vi "read All reg.vi"() -> ()   [LabVIEW 2010]
panel:
  out "x-y":u32=20388
  out "Array 2":i16[](array[numeric])=[5270, 1, 6098, 0, 2200, 2310, 7, 8, 8, 3, 3, 3, 3, 0, 0, -32000, 14, 30, 0, 0, 0, 0, 0, 0, 0, 0, 0, 0, 0, 0, 1, 0, 0, 0, 0, 0, 1, -32000, 0, 0, 0, 0, 1, 0, 0, 0, 0, 1, 0, 0, 0, -1, -999, -999, -999, 999, 999, 999, 90, 0, 0, 24, 0, 0, 0, -1, -999, -999, -999, 999, 999, 999, 90, 0, 24, 0, 0, 0, 0, 0, 14, 0, 0, 0, 0, 0, 10, 2, 1, 14, 0, 0, 0, 0, 0, 2, 14, 0, 0, 0, 0, 0, 2, 1, 1, 1, 1, 1, 1, 2, 14, 0, 0, 0, 0, 0, 2, 14, 0, 0, 0, 0, 0, 10, 2, 1, 14, 0, 0, 0, 0, 0, 2, 14, 0, 0, 0, 0, 0, 2, 14, 0, 0, 0, 0, 0, 2, 14, 0, 0, 0, 0, 0, 2, 0, 0, 0, 815, 0, 0, 0, 0, 0, 4, 0, 0, 815, 0, 0, 0, 0, 0, 4, 0, 0, 815, 0, 0, 0, 0, 0, 32, 1500, 32, 1500, 32, 1500, 1, 0, 0, 2, 0, 0, 0, 0, 0, 0, 0, 816, 0, 100, 0, 0, 0, 0, 0, 2, 0, 0, 0, 0, 0, 0, 0, 816, 0, 100, 0, 0, 1, 0, 100, 0, 0, 0, 100, 0, 0, 0, 0, 1, 0, 0, 0, 0, 0, 0, 0, 0, 0, 0, 0, 0, -1, -1, -1, -1, -1, -1, -1, -1, 1, 0, 0, 0, 1, 10, 0, 39, 239, 0, 1, 0, 0, 0, 0, 0, 0, 0, 0, 70, 52, 70, 52, 15, 16, 2, 4, 5, 22, 23, 24, 21, 14, 12, 13, 6, 7, 11, 10, 954, 12816, 13472, 0, 0, -32000, -32000, -32000, 50, 0, 21, 8, 24, 6, 28, 2011, 0, 1, 0, -19999, -19999, 9999, 9999, 0, 0, 0, 0, 0, 0, 0, 0, 0, 0, 0, 0, 0, 100, 30, 0, 0, -100, 30, 0, 0, 0, 0, 30, 10, 14, 0, 0, 0, 0, 0, 10, 2, 1, 14, 0, 0, 0, 0, 0, 2, 14, 0, 0, 0, 0, 0, 2, 14, 0, 0, 0, 0, 0, 2, 14, 0, 0, 0, 0, 0, 2, 14, 0, 0, 0, 0, 0, 10, 2, 1, 14, 0, 0, 0, 0, 0, 2, 14, 0, 0, 0, 0, 0, 2, 14, 0, 0, 0, 0, 0, 2, 14, 0, 0, 0, 0, 0, 2, 25, 0, 0, 0, 0, 0, 3, 25, 0, 0, 0, 0, 0, 3, 25, 0, 0, 0, 0, 0, 3, 25, 0, 0, 0, 0, 0, 3, 25, 0, 0, 0, 0, 0, 3, 25, 0, 0, 0, 0, 0, 3, 25, 0, 0, 0, 0, 0, 3, 25, 0, 0, 0, 0, 0, 3, 25, 0, 0, 0, 0, 0, 3, 25, 0, 0, 0, 0, 0, 3, 56, 55, 56, 55, 56, 56, 56, 78, 49, 32, 68, 73, 71, 73, 84, 32, 73, 78, 50, 32, 68, 73, 71, 73, 84, 32, 73, 78, 51, 32, 68, 73, 71, 73, 84, 32, 73, 78, 52, 32, 68, 73, 71, 73, 84, 32, 79, 85, 84, 49, 68, 73, 71, 73, 84, 32, 79, 85, 84, 50, 68, 73, 71, 73, 84, 32, 79, 85, 84, 51, 68, 73, 71, 73, 84, 32, 79, 85, 84, 52, 68, 73, 71, 73, 84, 32, 79, 85, 84, 53, 68, 73, 71, 73, 84, 32, 79, 85, 84, 54, 68, 73, 71, 73, 84, 32, 79, 85, 84, 55, 68, 73, 71, 73, 84, 32, 79, 85, 84, 56, 65, 76, 65, 82, 77, 49, 32, 32, 32, 32, 65, 76, 65, 82, 77, 50, 32, 32, 32, 32, 80, 82, 79, 70, 73, 76, 69, 49, 32, 32, 80, 82, 79, 70, 73, 76, 69, 50, 32, 32, 80, 82, 79, 70, 73, 76, 69, 51, 32, 32, 80, 82, 79, 70, 73, 76, 69, 52, 32, 32, 80, 82, 79, 70, 73, 76, 69, 53, 32, 32, 80, 82, 79, 70, 73, 76, 69, 54, 32, 32, 80, 82, 79, 70, 73, 76, 69, 55, 32, 32, 80, 82, 79, 70, 73, 76, 69, 56, 32, 32, 80, 82, 79, 70, 73, 76, 69, 57, 32, 32, 80, 82, 79, 70, 73, 76, 69, 49, 48, 32, 80, 82, 79, 70, 73, 76, 69, 49, 49, 32, 80, 82, 79, 70, 73, 76, 69, 49, 50, 32, 80, 82, 79, 70, 73, 76, 69, 49, 51, 32, 80, 82, 79, 70, 73, 76, 69, 49, 52, 32, 80, 82, 79, 70, 73, 76, 69, 49, 53, 32, 80, 82, 79, 70, 73, 76, 69, 49, 54, 32, 80, 82, 79, 70, 73, 76, 69, 49, 55, 32, 80, 82, 79, 70, 73, 76, 69, 49, 56, 32, 80, 82, 79, 70, 73, 76, 69, 49, 57, 32, 80, 82, 79, 70, 73, 76, 69, 50, 48, 32, 80, 82, 79, 70, 73, 76, 69, 50, 49, 32, 80, 82, 79, 70, 73, 76, 69, 50, 50, 32, 80, 82, 79, 70, 73, 76, 69, 50, 51, 32, 80, 82, 79, 70, 73, 76, 69, 50, 52, 32, 80, 82, 79, 70, 73, 76, 69, 50, 53, 32, 80, 82, 79, 70, 73, 76, 69, 50, 54, 32, 80, 82, 79, 70, 73, 76, 69, 50, 55, 32, 80, 82, 79, 70, 73, 76, 69, 50, 56, 32, 80, 82, 79, 70, 73, 76, 69, 50, 57, 32, 80, 82, 79, 70, 73, 76, 69, 51, 48, 32, 80, 82, 79, 70, 73, 76, 69, 51, 49, 32, 80, 82, 79, 70, 73, 76, 69, 51, 50, 32, 80, 82, 79, 70, 73, 76, 69, 51, 51, 32, 80, 82, 79, 70, 73, 76, 69, 51, 52, 32, 80, 82, 79, 70, 73, 76, 69, 51, 53, 32, 80, 82, 79, 70, 73, 76, 69, 51, 54, 32, 80, 82, 79, 70, 73, 76, 69, 51, 55, 32, 80, 82, 79, 70, 73, 76, 69, 51, 56, 32, 80, 82, 79, 70, 73, 76, 69, 51, 57, 32, 80, 82, 79, 70, 73, 76, 69, 52, 48, 32, 0, 0, -31300, -31300, -31300, -31300, -31300, -31300, -31300, -31300, -31300, -31300, -31300, -31300, -31300, -31300, -31300, -31300, -31300, -31300, -31300, -31300, -31300, -31300, -31300, -31300, -31300, -31300, -31300, -31300, -31300, -31300, -31300, -31300, -31300, -31300, -31300, -31300, -31300, -31300, -31300, -31300, -31300, -31300, 1, 17, 5, 1, 1, 1, 1, 1, 1, 1, 1, 0, 0, 0, 0, 0, 0, 0, 0, 0, 0, 0, 0, 0, 0, 5, 1, 1, 15, 75, 75, 77, 69, 83, 83, 65, 71, 69, 32, 49, 32, 32, 32, 32, 32, 32, 32, 32, 32, 77, 69, 83, 83, 65, 71, 69, 32, 50, 32, 32, 32, 32, 32, 32, 32, 32, 32, 77, 69, 83, 83, 65, 71, 69, 32, 51, 32, 32, 32, 32, 32, 32, 32, 32, 32, 77, 69, 83, 83, 65, 71, 69, 32, 52, 32, 32, 32, 32, 32, 32, 32, 32, 32, 0, 2, 2, 2]
  out "Data":i16[](array[numeric])
  out "error out":errorcluster
  out "Numeric":i32=93
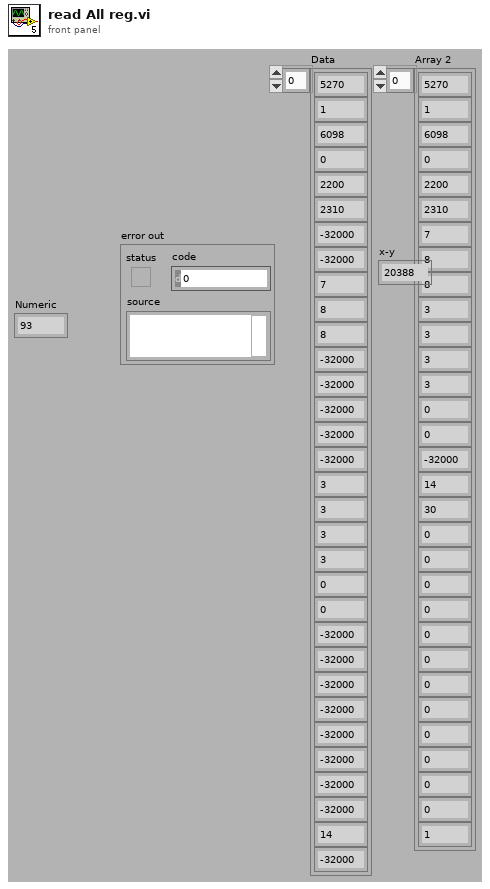
[diagram p1: front panel]
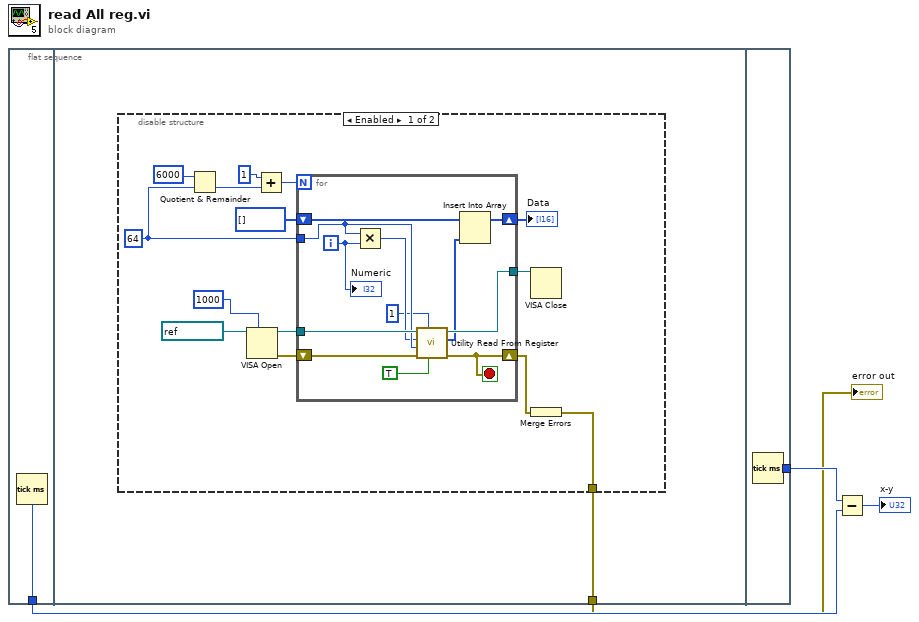
[diagram p0: block diagram]
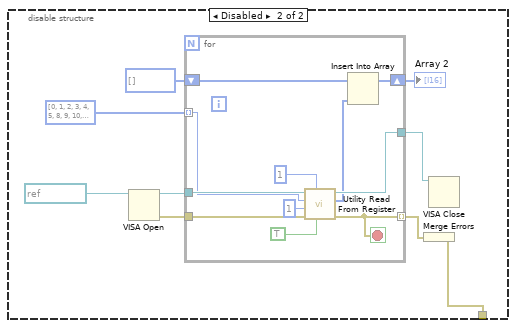
[diagram p2: hidden frame]
diagram:
  n1 = flat-sequence {
    tunnel: [w5] -> w3
    tunnel: [w6] -> w1
    tunnel: [w53] -> w4
    frame #0 {
      n2 = Tick Count (ms)() -> (millisecond timer value=w5:u32)
    }
    frame #1 {
      n3 = disable-structure shown="Enabled" {
        disable-tunnel: [w7 w33] -> w6
        frame Enabled {
          w15 = u16 64 ("Num Of Reg (1)")
          n4 = Quotient & Remainder(x=u16 6000, y=w15) -> (floor(x/y)=w18:u16)  [unwired: 1 out]
          n5 = VISA Open(timeout (0)=u32 1000 ("VISA Open timeout (0)"), VISA resource name=refnum<visa-resource-name> "COM1") -> (VISA resource name=w20:refnum<visa-resource-name>, error out=w12:errorcluster)  [unwired: 3 in]
          n6 = Add(x=u16 1, y=w18) -> (x+y=w17:u16)
          n7 = for {
            N: w17 -> [_]
            tunnel: w20 -> [w31]
            tunnel: w15 -> [w29]
            tunnel: [w25] -> w11
            shift-right: [w23] -> w8
            shift-left: i16[] [] -> [w22]
            shift-right: [w21] -> w10
            shift-left: w12 -> [w26]
            i -> [w30]
            stop <- w21 stop-if-true
            n8 = Multiply(x=w29, y=w30) -> (x*y=w28:i32)
            n9 = call "Utility Read From Register.vi"("Direct Action?"=TRUE, "Unit Address (1)"=u8 1, "error in (no error)"=w26, "Num Of Reg (1)"=w29, "Register Address (0)"=w28, "VISA resource name"=w31) -> ("error out"=w21:errorcluster, "Data"=w24:i16[], "VISA resource name out"=w25:refnum<visa-resource-name>)  [unwired: 3 in]
            n10 = Insert Into Array(array=w22, new element=w24) -> (w23:i16[])  [unwired: 1 in]
            "Numeric" <- w30
          }
          "Data" <- w8
          n11 = VISA Close(VISA resource name=w11) -> ()  [unwired: 1 in, 1 out]
          n12 = Merge Errors(w10) -> (w7:errorcluster)
        }
        frame Disabled {
          n13 = VISA Open(VISA resource name=refnum<visa-resource-name> "COM1") -> (VISA resource name=w34:refnum<visa-resource-name>, error out=w35:errorcluster)  [unwired: 4 in]
          n14 = for {
            tunnel: [w45] -> w37 mode=indexing
            tunnel: w34 -> [w44]
            tunnel: w35 -> [w50]
            tunnel: [w49] -> w36
            shift-right: [w47] -> w40
            shift-left: i16[] [] -> [w46]
            tunnel: i64[] [0, 1, 2, 3, 4, 5, 8, 9, 10, 16, 17, 18, 19, 20, 21, 25, 30, 100, 101, 102, 103, 104, 105, 106, 107, 108, 109, 111, 115, 200, 201, 204, 205, 206, 207, 210, 213, 216, 217, 218, 219, 222, 225, 228, 229, 230, 231, 237, 241, 242, 243, 300, 302, 302, 302, 303, 303, 303, 304, 305, 305, 308, 311, 312, 313, 319, 321, 321, 321, 322, 322, 322, 323, 324, 327, 330, 331, 332, 343, 349, 500, 501, 502, 503, 504, 505, 506, 507, 509, 510, 511, 512, 513, 514, 515, 517, 520, 521, 522, 523, 524, 525, 527, 530, 531, 532, 533, 534, 535, 537, 540, 541, 542, 543, 544, 545, 547, 550, 551, 552, 553, 554, 555, 556, 557, 559, 560, 561, 562, 563, 564, 565, 567, 570, 571, 572, 573, 574, 575, 577, 580, 581, 582, 583, 584, 585, 587, 590, 591, 592, 593, 594, 595, 597, 600, 601, 602, 603, 604, 605, 606, 607, 608, 610, 611, 612, 613, 614, 615, 616, 617, 618, 620, 621, 622, 623, 624, 625, 626, 627, 628, 680, 681, 682, 683, 684, 685, 700, 701, 702, 703, 704, 705, 706, 707, 708, 709, 710, 711, 712, 714, 715, 716, 717, 718, 719, 720, 721, 722, 723, 724, 725, 726, 727, 728, 729, 731, 732, 733, 734, 735, 748, 749, 751, 752, 765, 766, 836, 837, 900, 901, 903, 904, 906, 907, 1060, 1061, 1062, 1063, 1064, 1065, 1066, 1067, 1075, 1076, 1077, 1078, 1079, 1080, 1081, 1082, 1205, 1206, 1209, 1210, 1212, 1213, 1217, 1218, 1219, 1220, 1221, 1300, 1302, 1303, 1306, 1307, 1308, 1309, 1315, 1330, 1331, 1332, 1333, 1400, 1401, 1402, 1403, 1404, 1405, 1406, 1407, 1408, 1409, 1410, 1411, 1412, 1413, 1414, 1415, 1500, 1501, 1504, 1505, 1506, 1512, 1513, 1514, 1515, 1902, 1916, 1917, 1918, 1919, 1920, 1921, 1922, 1923, 1925, 1926, 1926, 1927, 1927, 2000, 2001, 2010, 2011, 2020, 2021, 2030, 2031, 2040, 2041, 2046, 2050, 2051, 2052, 2054, 2060, 2061, 2062, 2064, 2070, 2071, 2072, 2073, 2074, 2075, 2500, 2501, 2502, 2503, 2504, 2505, 2506, 2507, 2509, 2510, 2511, 2512, 2513, 2514, 2515, 2517, 2520, 2521, 2522, 2523, 2524, 2525, 2527, 2530, 2531, 2532, 2533, 2534, 2535, 2537, 2540, 2541, 2542, 2543, 2544, 2545, 2547, 2550, 2551, 2552, 2553, 2554, 2555, 2556, 2557, 2559, 2560, 2561, 2562, 2563, 2564, 2565, 2567, 2570, 2571, 2572, 2573, 2574, 2575, 2577, 2580, 2581, 2582, 2583, 2584, 2585, 2587, 2590, 2591, 2592, 2593, 2594, 2595, 2597, 2600, 2601, 2602, 2603, 2604, 2605, 2607, 2610, 2611, 2612, 2613, 2614, 2615, 2617, 2620, 2621, 2622, 2623, 2624, 2625, 2627, 2630, 2631, 2632, 2633, 2634, 2635, 2637, 2640, 2641, 2642, 2643, 2644, 2645, 2647, 2650, 2651, 2652, 2653, 2654, 2655, 2657, 2660, 2661, 2662, 2663, 2664, 2665, 2667, 2670, 2671, 2672, 2673, 2674, 2675, 2677, 2680, 2681, 2682, 2683, 2684, 2685, 2687, 2690, 2691, 2692, 2693, 2694, 2695, 2697, 3000, 3001, 3002, 3003, 3004, 3005, 3006, 3007, 3008, 3009, 3010, 3011, 3012, 3013, 3014, 3015, 3016, 3017, 3018, 3019, 3020, 3021, 3022, 3023, 3024, 3025, 3026, 3027, 3028, 3029, 3030, 3031, 3032, 3033, 3034, 3035, 3036, 3037, 3038, 3039, 3100, 3101, 3102, 3103, 3104, 3105, 3106, 3107, 3108, 3109, 3110, 3111, 3112, 3113, 3114, 3115, 3116, 3117, 3118, 3119, 3120, 3121, 3122, 3123, 3124, 3125, 3126, 3127, 3128, 3129, 3130, 3131, 3132, 3133, 3134, 3135, 3136, 3137, 3138, 3139, 3140, 3141, 3142, 3143, 3144, 3145, 3146, 3147, 3148, 3149, 3150, 3151, 3152, 3153, 3154, 3155, 3156, 3157, 3158, 3159, 3160, 3161, 3162, 3163, 3164, 3165, 3166, 3167, 3168, 3169, 3170, 3171, 3172, 3173, 3174, 3175, 3176, 3177, 3178, 3179, 3200, 3201, 3202, 3203, 3204, 3205, 3206, 3207, 3208, 3209, 3210, 3211, 3212, 3213, 3214, 3215, 3216, 3217, 3218, 3219, 3500, 3501, 3502, 3503, 3504, 3505, 3506, 3507, 3508, 3509, 3510, 3511, 3512, 3513, 3514, 3515, 3516, 3517, 3518, 3519, 3520, 3521, 3522, 3523, 3524, 3525, 3526, 3527, 3528, 3529, 3530, 3531, 3532, 3533, 3534, 3535, 3536, 3537, 3538, 3539, 3540, 3541, 3542, 3543, 3544, 3545, 3546, 3547, 3548, 3549, 3550, 3551, 3552, 3553, 3554, 3555, 3556, 3557, 3558, 3559, 3560, 3561, 3562, 3563, 3564, 3565, 3566, 3567, 3568, 3569, 3570, 3571, 3572, 3573, 3574, 3575, 3576, 3577, 3578, 3579, 3580, 3581, 3582, 3583, 3584, 3585, 3586, 3587, 3588, 3589, 3590, 3591, 3592, 3593, 3594, 3595, 3596, 3597, 3598, 3599, 3600, 3601, 3602, 3603, 3604, 3605, 3606, 3607, 3608, 3609, 3610, 3611, 3612, 3613, 3614, 3615, 3616, 3617, 3618, 3619, 3620, 3621, 3622, 3623, 3624, 3625, 3626, 3627, 3628, 3629, 3630, 3631, 3632, 3633, 3634, 3635, 3636, 3637, 3638, 3639, 3640, 3641, 3642, 3643, 3644, 3645, 3646, 3647, 3648, 3649, 3650, 3651, 3652, 3653, 3654, 3655, 3656, 3657, 3658, 3659, 3660, 3661, 3662, 3663, 3664, 3665, 3666, 3667, 3668, 3669, 3670, 3671, 3672, 3673, 3674, 3675, 3676, 3677, 3678, 3679, 3680, 3681, 3682, 3683, 3684, 3685, 3686, 3687, 3688, 3689, 3690, 3691, 3692, 3693, 3694, 3695, 3696, 3697, 3698, 3699, 3700, 3701, 3702, 3703, 3704, 3705, 3706, 3707, 3708, 3709, 3710, 3711, 3712, 3713, 3714, 3715, 3716, 3717, 3718, 3719, 3720, 3721, 3722, 3723, 3724, 3725, 3726, 3727, 3728, 3729, 3730, 3731, 3732, 3733, 3734, 3735, 3736, 3737, 3738, 3739, 3740, 3741, 3742, 3743, 3744, 3745, 3746, 3747, 3748, 3749, 3750, 3751, 3752, 3753, 3754, 3755, 3756, 3757, 3758, 3759, 3760, 3761, 3762, 3763, 3764, 3765, 3766, 3767, 3768, 3769, 3770, 3771, 3772, 3773, 3774, 3775, 3776, 3777, 3778, 3779, 3780, 3781, 3782, 3783, 3784, 3785, 3786, 3787, 3788, 3789, 3790, 3791, 3792, 3793, 3794, 3795, 3796, 3797, 3798, 3799, 3800, 3801, 3802, 3803, 3804, 3805, 3806, 3807, 3808, 3809, 3810, 3811, 3812, 3813, 3814, 3815, 3816, 3817, 3818, 3819, 3820, 3821, 3822, 3823, 3824, 3825, 3826, 3827, 3828, 3829, 3830, 3831, 3832, 3833, 3834, 3835, 3836, 3837, 3838, 3839, 3840, 3841, 3842, 3843, 3844, 3845, 3846, 3847, 3848, 3849, 3850, 3851, 3852, 3853, 3854, 3855, 3856, 3857, 3858, 3859, 3860, 3861, 3862, 3863, 3864, 3865, 3866, 3867, 3868, 3869, 3870, 3871, 3872, 3873, 3874, 3875, 3876, 3877, 3878, 3879, 3880, 3881, 3882, 3883, 3884, 3885, 3886, 3887, 3888, 3889, 3890, 3891, 3892, 3893, 3894, 3895, 3896, 3897, 3898, 3899, 4000, 4001, 4002, 4003, 4004, 4005, 4006, 4007, 4008, 4009, 4010, 4011, 4012, 4013, 4014, 4015, 4016, 4021, 4022, 4023, 4024, 4025, 4026, 4030, 4031, 4032, 4033, 4034, 4035, 4036, 4037, 4043, 4044, 4045, 4046, 4047, 4048, 4049, 4050, 4051, 4052, 4060, 4061, 4062, 4100, 4101, 4102, 4103, 4104, 4105, 4106, 4107, 4108, 4109, 4110, 4111, 4112, 4113, 4114, 4115, 4116, 4117, 4118, 4119, 4120, 4121, 4122, 4123, 4124, 4125, 4126, 4127, 4128, 4129, 4130, 4501, 4502, 4503, 4504, 4505, 4506, 4507, 4508, 4509, 4510, 4511, 4512, 4513, 4514, 4515, 4516, 4517, 4518, 4521, 4522, 4523, 4524, 4525, 4526, 4527, 4528, 4529, 4530, 4531, 4532, 4533, 4534, 4535, 4536, 4537, 4538, 4541, 4542, 4543, 4544, 4545, 4546, 4547, 4548, 4549, 4550, 4551, 4552, 4553, 4554, 4555, 4556, 4557, 4558, 4561, 4562, 4563, 4564, 4565, 4566, 4567, 4568, 4569, 4570, 4571, 4572, 4573, 4574, 4575, 4576, 4577, 4578, 5500, 5501, 5502, 5503] ("subarray") -> [w42] mode=indexing
            stop <- w45 stop-if-true
            n15 = call "Utility Read From Register.vi"("Direct Action?"=TRUE, "Unit Address (1)"=u8 1, "error in (no error)"=w50, "Num Of Reg (1)"=u16 1, "Register Address (0)"=w42, "VISA resource name"=w44) -> ("error out"=w45:errorcluster, "Data"=w48:i16[], "VISA resource name out"=w49:refnum<visa-resource-name>)  [unwired: 3 in]
            n16 = Insert Into Array(array=w46, new element=w48) -> (w47:i16[])  [unwired: 1 in]
          }
          "Array 2" <- w40
          n17 = Merge Errors(w37) -> (w33:errorcluster)
          n18 = VISA Close(VISA resource name=w36) -> ()  [unwired: 1 in, 1 out]
        }
      }
    }
    frame #2 {
      n19 = Tick Count (ms)() -> (millisecond timer value=w53:u32)
    }
  }
  n20 = Subtract(x=w4, y=w3) -> (x-y=→"x-y":u32)
  "error out" <- w1
